vi "TCL Log Event to Disk.vi"(0 "event file":path, 1 "event":string[](array[string]), 7 "signals":cluster{"name":string, "values":string[]}[](array[cluster]), 9 "primary key":dbl, 11 "error in (no error)":errorcluster) -> (15 "error out":errorcluster)   [LabVIEW 2010]
uses:
  <vilib>/Utility/file.llb/Write To Spreadsheet File (string).vi
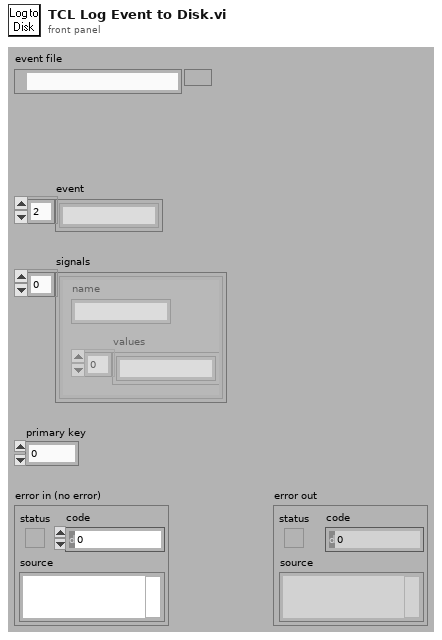
[diagram p1: front panel]
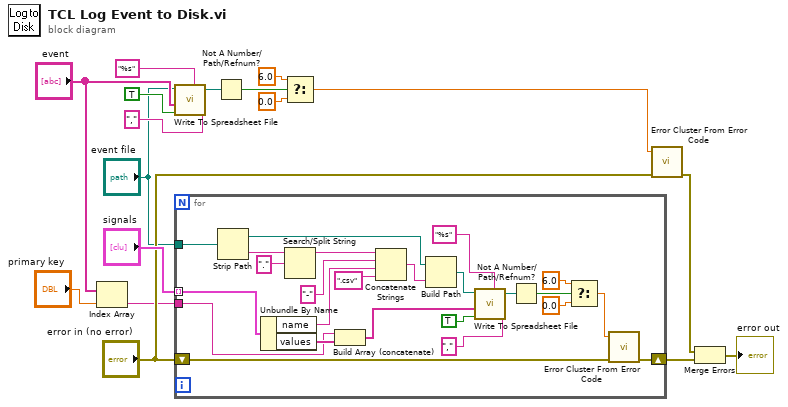
[diagram p0: block diagram]
diagram:
  n1 = Index Array(array="event", index="primary key") -> (element=w2:string)
  n2 = call-poly <vilib>:"Write To Spreadsheet File.vi"("delimiter (\\t)"="," ("delimiter (\\t)"), "format (%s)"="%s" ("format (%.3f)"), "append to file? (new file:F)"=TRUE, "1D data"="event", "file path (dialog if empty)"="event file") -> ("new file path (Not A Path if cancelled)"=w10:path)  [unwired: 3 in]
  n3 = for {
    tunnel: "signals" -> [w41] mode=indexing
    tunnel: "event file" -> [w40]
    shift-right: [w30] -> w6
    shift-left: "error in (no error)" -> [w31]
    tunnel: w2 -> [w22]
    n4 = Strip Path(path=w40) -> (stripped path=w21:path, name=w20:string)
    n5 = Unbundle By Name(w41) -> ("name"=w39:string, "values"=w24:string[])
    n6 = Search/Split String(string=w20, search string/char (-)=".") -> (substring before match=w18:string)  [unwired: 1 in, 2 out]
    n7 = Build Array (concatenate)(w22, w24) -> (w23:string[])
    n8 = Concatenate Strings(w18, "-" ("string"), w39, ".csv" ("string")) -> (w38:string)
    n9 = Build Path(base path=w21, name or relative path=w38) -> (appended path=w33:path)
    n10 = call-poly <vilib>:"Write To Spreadsheet File.vi"("delimiter (\\t)"="," ("delimiter (\\t)"), "format (%s)"="%s" ("format (%.3f)"), "append to file? (new file:F)"=TRUE, "1D data"=w23, "file path (dialog if empty)"=w33) -> ("new file path (Not A Path if cancelled)"=w29:path)  [unwired: 3 in]
    n11 = Not A Number/Path/Refnum?(number/path/refnum=w29) -> (NaN/Path/Refnum?=w28:bool)
    n12 = Select(t=6.0, s=w28, f=0.0) -> (s? t:f=w25:dbl)
    n13 = call <vilib>:"Error Cluster From Error Code.vi"("error in (no error)"=w31, "error code (0)"=w25) -> ("error out"=w30:errorcluster)  [unwired: 7 in]
  }
  n14 = Not A Number/Path/Refnum?(number/path/refnum=w10) -> (NaN/Path/Refnum?=w13:bool)
  n15 = Select(t=6.0, s=w13, f=0.0) -> (s? t:f=w9:dbl)
  n16 = call <vilib>:"Error Cluster From Error Code.vi"("error in (no error)"="error in (no error)", "error code (0)"=w9) -> ("error out"=w7:errorcluster)  [unwired: 7 in]
  n17 = Merge Errors(w7, w6) -> (→"error out":errorcluster)
